vi "Open.vi"(8 "error in (no error)":errorcluster, 10 "address":string, 11 "Instrument.AFM_DLog in":refnum<class "Instrument.AFM_DLog.lvclass">) -> (0 "error out":errorcluster, 3 "Instrument.AFM_DLog out":refnum<class "Instrument.AFM_DLog.lvclass">)   [LabVIEW 2019, in "Instrument.AFM_DLog.lvclass"]
uses:
  Instrument.AFM_DLog.lvclass
  C:/Program Files (x86)/National Instruments/LabVIEW 2019/user.lib/LevyLab/Instrument Framework/Instrument/Instrument.lvclass
  <userlib>/LevyLab/Instrument Framework/Instrument Types/SCPI/Instrument.SCPI.lvclass
  <userlib>/LevyLab/Instrument Framework/Instrument/Instrument.lvclass
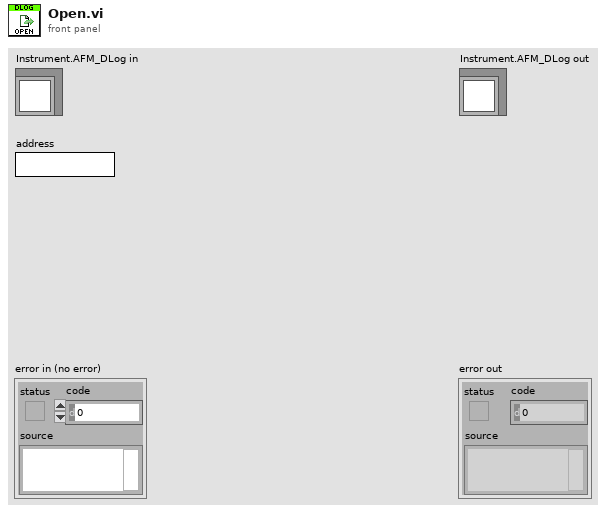
[diagram p1: front panel]
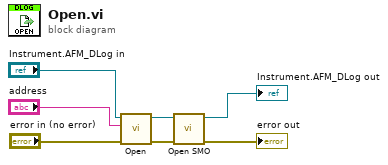
[diagram p0: block diagram]
diagram:
  n1 = call-parent "Open.vi"("error in (no error)"="error in (no error)", "address"="address", "Instrument in"="Instrument.AFM_DLog in") -> ("error out"=w4:errorcluster, "Instrument out"=w3:refnum<class "Instrument.AFM_DLog.lvclass">)  [unwired: 7 in]
  n2 = call <userlib>:"Open SMO.vi"("error in (no error)"=w4, "Instrument in"=w3) -> ("error out"=→"error out":errorcluster, "Instrument out"=→"Instrument.AFM_DLog out":refnum<class "Instrument.AFM_DLog.lvclass">)  [unwired: 8 in]
